vi "Excel Export Data.vi"(6 "Comments":string="Comment Thread", 7 "Channel Names":string[](array[string]), 8 "error in (no error)":errorcluster, 9 "Raw Data":dbl[][][](array[numeric]), 10 "Processed Data":dbl[][](array[numeric]), 11 "File Name":path) -> (0 "error out":errorcluster)   [LabVIEW 2012]
doc: "Writes Arrays to individual sheets in one Excel Workbook. The same Comments box and Channel Names are written to each sheet.\n\nData passed to this should be arranged in columns."
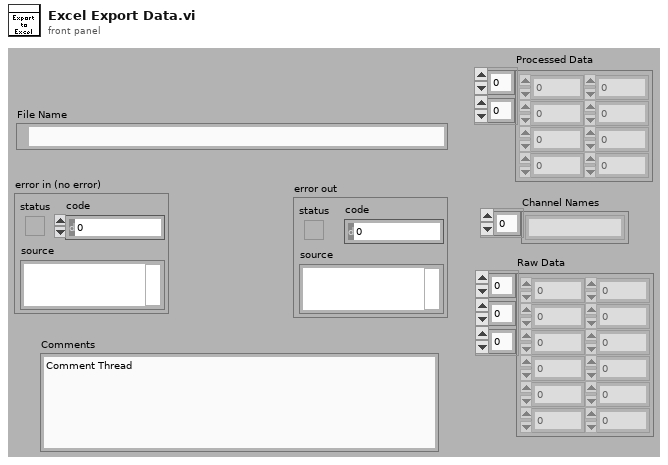
[diagram p1: front panel]
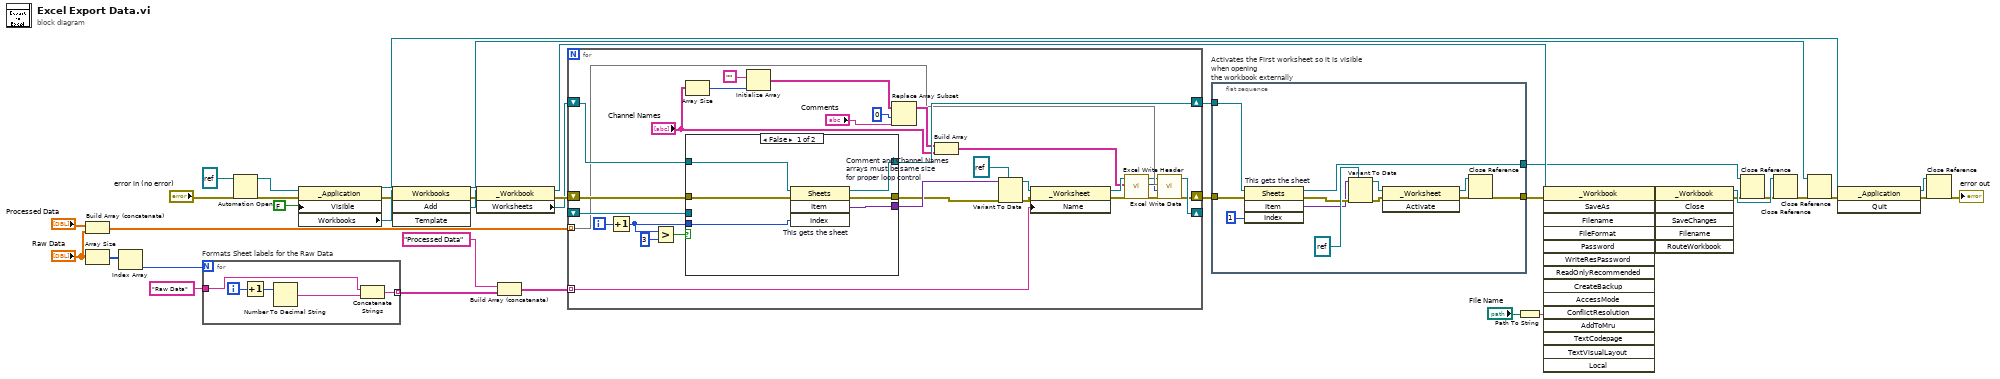
[diagram p0: block diagram]
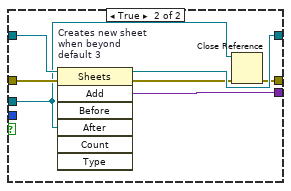
[diagram p2: hidden frame]
diagram:
  n1 = Build Array (concatenate)("Processed Data", "Raw Data") -> (w21:dbl[][][])
  n2 = Array Size(array="Raw Data") -> (size(s)=w18:i32[])
  n3 = Index Array(array=w18) -> (element=w17:i32)  [unwired: 1 in]
  n4 = for "Formats Sheet labels for the Raw Data" {
    N: w17 -> [_]
    tunnel: "Raw Data" -> [w44]
    tunnel: [w42] -> w8 mode=indexing
    i -> [w41]
    n5 = Increment(x=w41) -> (x+1=w40:i32)
    n6 = Number To Decimal String(number=w40) -> (decimal integer string=w43:string)  [unwired: 1 in]
    n7 = Concatenate Strings(w44, w43) -> (w42:string)
  }
  n8 = Automation Open(error in (no error)="error in (no error)", Automation Refnum=refnum<k7> refnum ("Excel Application")) -> (Automation Refnum=w7:refnum<k7>, error out=w1:errorcluster)  [unwired: 2 in]
  n9 = property class="_Application"(reference=w7, error in=w1, "Visible"=FALSE) -> (reference out=w28:refnum<k7>, error out=w34:errorcluster, "Workbooks"=w36:refnum<k7>)
  n10 = invoke class="Workbooks" method="Add"(reference=w36, error in=w34) -> (reference out=w15:refnum<k7>, error out=w33:errorcluster, "Add"=w35:refnum<k7>)  [unwired: 2 in, 1 out]
  n11 = property class="_Workbook"(reference=w35, error in=w33) -> (reference out=w31:refnum<k7>, error out=w32:errorcluster, "Worksheets"=w20:refnum<k7>)
  n12 = Build Array (concatenate)("Processed Data", w8) -> (w19:string[])
  n13 = for {
    shift-right: [w45] -> w3
    shift-left: w32 -> [w71]
    shift-right: [w68] -> w5
    shift-left: w20 -> [w74]
    tunnel: w21 -> [w50] mode=indexing
    tunnel: w19 -> [w66] mode=indexing
    shift-right: [w46] -> _
    shift-left: _ -> [w61]
    i -> [w69]
    n14 = Increment(x=w69) -> (x+1=w63:i32)
    n15 = Greater?(x=w63, y=3) -> (0:w64:bool)
    n16 = Array Size(array="Channel Names") -> (size(s)=w58:i32)
    n17 = case shown="False" w64 {
      tunnel: w74 -> [w80 w87]
      tunnel: [w79 w85] -> w73
      tunnel: w71 -> [w78 w86]
      tunnel: [w77 w82] -> w70
      tunnel: w63 -> [w76 _]
      tunnel: [w75 w84] -> w68
      tunnel: w61 -> [_ w81]
      frame False {
        n18 = invoke on="This gets the sheet" class="Sheets" method="Item"(reference=w80, error in=w78, "Index"=w76) -> (reference out=w75:refnum<k7>, error out=w77:errorcluster, "Item"=w79:variant)  [unwired: 1 in, 1 out]
      }
      frame True {
        n19 = invoke on="Creates new sheet\nwhen beyond\ndefault 3" class="Sheets" method="Add"(reference=w87, error in=w86, "After"=w81) -> (reference out=w84:refnum<k7>, error out=w83:errorcluster, "Add"=w85:variant)  [unwired: 4 in, 4 out]
        n20 = Close Reference(reference=w81, error in (no error)=w83) -> (error out=w82:errorcluster)
      }
    }
    n21 = Initialize Array("", w58) -> (w55:string[])
    n22 = Replace Array Subset(array=w55, new element="Comments", index=0) -> (w54:string[])
    n23 = Build Array "Comment and Channel Names\narrays must be same size\nfor proper loop control"(w54, "Channel Names") -> (w51:string[][])
    n24 = Variant To Data(error in=w70, type=refnum<k7> refnum ("reference"), Variant=w73) -> (data=w67:refnum<k7>, error out=w65:errorcluster)
    n25 = property class="_Worksheet"(reference=w67, error in=w65, "Name"=w66) -> (reference out=w53:refnum<k7>, error out=w52:errorcluster)
    n26 = call "Excel Write Header.vi"("error in"=w52, "Header Data"=w51, "_Worksheet In"=w53) -> ("error out"=w48:errorcluster, "Header Size"=w49:i32, "_Worksheet Out"=w47:refnum<k7>)  [unwired: 6 in]
    n27 = call "Excel Write Data.vi"("error in"=w48, "Header Size"=w49, "Data"=w50, "_Worksheet In"=w47) -> ("error out"=w45:errorcluster, "_Worksheet Out"=w46:refnum<k7>)  [unwired: 6 in]
  }
  n28 = flat-sequence "Activates the First worksheet so it is visible when opening \nthe workbook externally" {
    tunnel: w5 -> [w97]
    tunnel: [w96] -> w4
    tunnel: w3 -> [w95]
    tunnel: [w91] -> w2
    frame #0 {
      n29 = invoke on="This gets the sheet" class="Sheets" method="Item"(reference=w97, error in=w95, "Index"=1) -> (reference out=w96:refnum<k7>, error out=w94:errorcluster, "Item"=w90:variant)  [unwired: 1 in, 1 out]
      n30 = Variant To Data(error in=w94, type=refnum<k7> refnum ("reference"), Variant=w90) -> (data=w89:refnum<k7>, error out=w93:errorcluster)
      n31 = invoke class="_Worksheet" method="Activate"(reference=w89, error in=w93) -> (reference out=w88:refnum<k7>, error out=w92:errorcluster)  [unwired: 1 in, 1 out]
      n32 = Close Reference(reference=w88, error in (no error)=w92) -> (error out=w91:errorcluster)
    }
  }
  n33 = Path To String(path="File Name") -> (string=w22:string)
  n34 = invoke class="_Workbook" method="SaveAs"(reference=w31, error in=w2, "Filename"=w22) -> (reference out=w30:refnum<k7>, error out=w29:errorcluster)  [unwired: 12 in, 13 out]
  n35 = invoke class="_Workbook" method="Close"(reference=w30, error in=w29) -> (reference out=w27:refnum<k7>, error out=w13:errorcluster)  [unwired: 4 in, 4 out]
  n36 = Close Reference(reference=w4, error in (no error)=w13) -> (error out=w12:errorcluster)
  n37 = Close Reference(reference=w27, error in (no error)=w12) -> (error out=w14:errorcluster)
  n38 = Close Reference(reference=w15, error in (no error)=w14) -> (error out=w6:errorcluster)
  n39 = invoke class="_Application" method="Quit"(reference=w28, error in=w6) -> (reference out=w25:refnum<k7>, error out=w26:errorcluster)  [unwired: 1 in, 1 out]
  n40 = Close Reference(reference=w25, error in (no error)=w26) -> (error out=→"error out":errorcluster)
